vi "CSVtoLabViewV2.0.vi"(10 "Sensor Unit Conversion":dbl, 11 "file path (dialog if empty)":path) -> (3 "Trajectory Point Array":T1[](array[typedef]))   [LabVIEW 2017]
uses:
  TrajectoryPointClusterV2.0.ctl
  <vilib>/Utility/file.llb/Read Delimited Spreadsheet (string).vi
  <vilib>/Utility/file.llb/Read Delimited Spreadsheet (DBL).vi
panel:
  out "Header":string[](array[string])
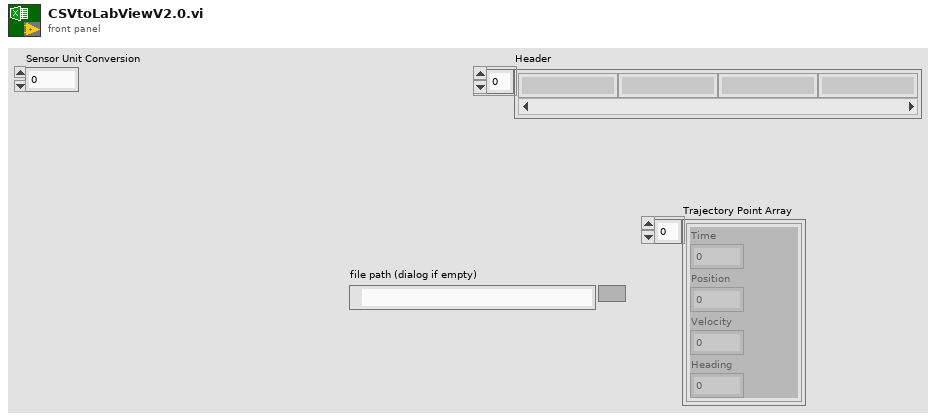
[diagram p1: front panel]
types:
  T1 = typedef "TrajectoryPointClusterV2.0.ctl" = cluster{"Position":dbl, "Velocity":dbl, "Heading":dbl, "Time":dbl}
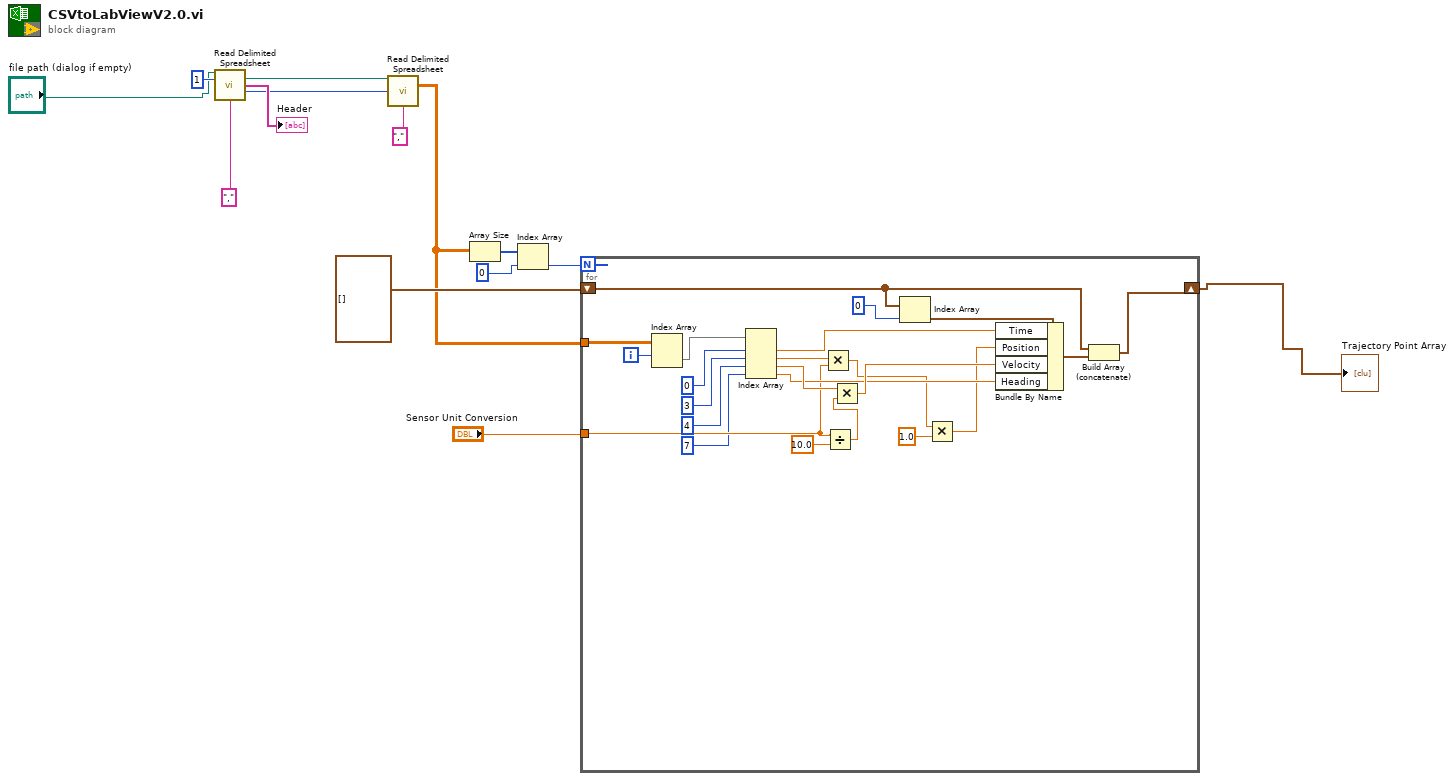
[diagram p0: block diagram]
diagram:
  n1 = call-poly <vilib>:"Read Delimited Spreadsheet.vi"("file path (dialog if empty)"="file path (dialog if empty)", "number of rows (all:-1)"=1, "delimiter (\\t)"="," ("delimiter (\\t)")) -> ("new file path (Not A Path if cancelled)"=w5:path, "first row"=→"Header":string[], "mark after read (chars.)"=w7:i32)  [unwired: 7 in, 3 out]
  n2 = call-poly <vilib>:"Read Delimited Spreadsheet.vi"("file path (dialog if empty)"=w5, "start of read offset (chars.:0)"=w7, "delimiter (\\t)"="," ("delimiter (\\t)")) -> ("all rows"=w4:dbl[][])  [unwired: 7 in, 5 out]
  n3 = Array Size(array=w4) -> (size(s)=w14:i32[])
  n4 = Index Array(array=w14, index=0) -> (element=w12:i32)
  n5 = for {
    N: w12 -> [_]
    shift-right: [w36] -> w1
    shift-left: T1[] [] -> [w17]
    tunnel: w4 -> [w35]
    tunnel: "Sensor Unit Conversion" -> [w28]
    i -> [w18]
    n6 = Index Array(array=w35, index (row)=w18) -> (element=w34:dbl[])  [unwired: 1 in]
    n7 = Index Array(array=w34, index #1=0 ("index"), index #2=3 ("index"), index #3=4 ("index"), index #4=7 ("index")) -> (element #1=w30:dbl, element #2=w33:dbl, element #3=w32:dbl, element #4=w29:dbl)
    n8 = Multiply(x=w33, y=w28) -> (x*y=w25:dbl)
    n9 = Divide(x=w28, y=10.0) -> (x/y=w26:dbl)
    n10 = Multiply(x=w32, y=w26) -> (x*y=w31:dbl)
    n11 = Index Array(array=w17, index=0) -> (element=w15:T1)
    n12 = Multiply(x=w25, y=1.0) -> (x*y=w23:dbl)
    n13 = Bundle By Name(cluster=w15, "Time"=w30, "Position"=w23, "Velocity"=w31, "Heading"=w29) -> (w37:T1)
    n14 = Build Array (concatenate)(w17, w37) -> (w36:T1[])
  }
  "Trajectory Point Array" <- w1
